vi "SSC Relay Control Single Action Single Site.vi"(0 "SSC Relay in":T1[](array[typedef]), 1 "Site":i32, 5 "Relay Action":T3=21 items=["Open Relay"=20, "Close Relay"=21], 7 "Settling Time (s)":dbl format="%#_12p", 9 "Sites":i32[](array[numeric]), 11 "error in":errorcluster) -> (4 "SSC Relay out":T1[](array[typedef]), 8 "Completed Relay Operations":T2[](array[typedef]) {"Desired State" items=["Open Relay"=20, "Close Relay"=21]}, 15 "error out":errorcluster)   [LabVIEW 2019]
doc: "Performs the specified relay action on all Relays associated with the specified site that are configured in the SSC Relay session. The function will then wait a specified amount of time if the Settling Time (s) input is wired."
uses:
  SSC Relay.ctl
  <instrlib>/niSwitch/niSwitch.llb/niSwitch Relay Action.ctl
  SubVIs/TSM Relay Completed Operations.ctl
  SSC Relay Control Core.vi
  Single SSC Relay NI-Switch Control.vi
  Single SSC Relay Fill Additional Error info.vi
  SSC Relay Expand Action Array to All Sessions.vi
  <vilib>/Utility/error.llb/Error Cluster From Error Code.vi
  <instrlib>/niSwitch/niSwitch.llb/niSwitch Get Relay Position.vi
  <instrlib>/niSwitch/niSwitch.llb/niSwitch Relay Control.vi
  <vilib>/Utility/High Resolution Polling Wait.vi
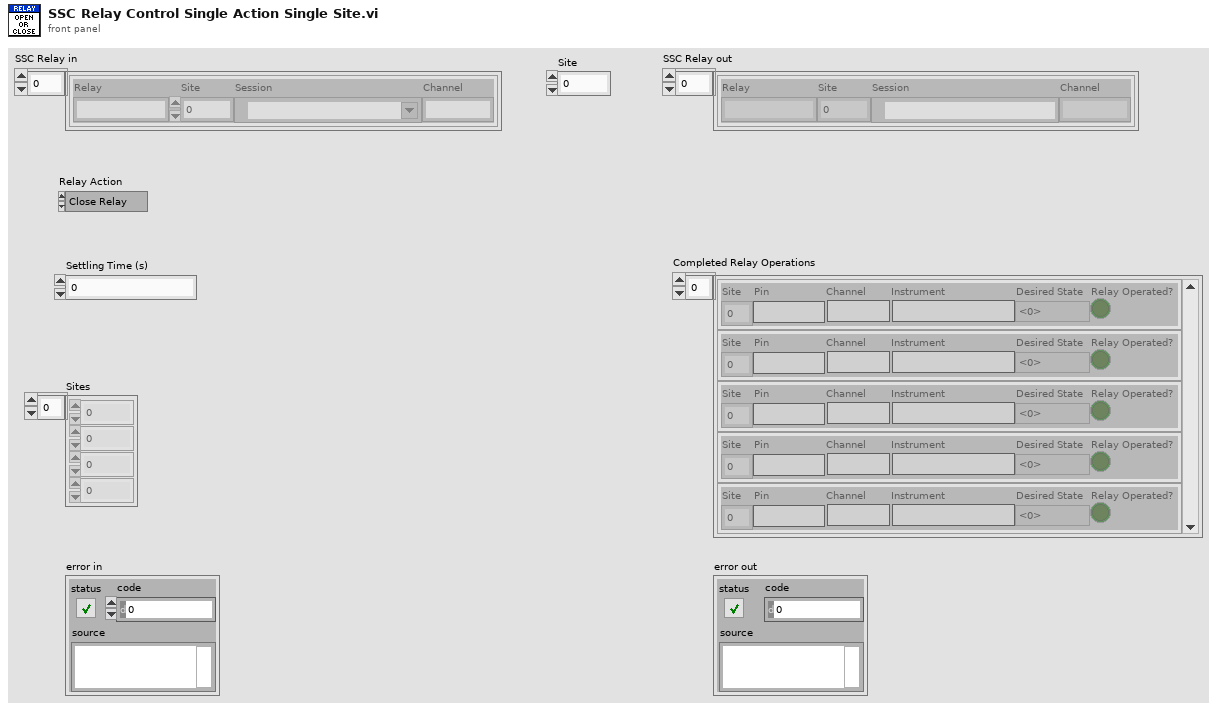
[diagram p1: front panel]
types:
  T1 = typedef "SSC Relay.ctl" = cluster{"Relay":string, "Site":i32, "Session":refnum<k15>, "Channel":string}
  T2 = typedef "TSM Relay Completed Operations.ctl" = cluster{"Site":i32, "Pin":string, "Channel":string, "Instrument":string, "Desired State":T3, "Relay Operated?":bool}
  T3 = typedef "niSwitch Relay Action.ctl" = i32
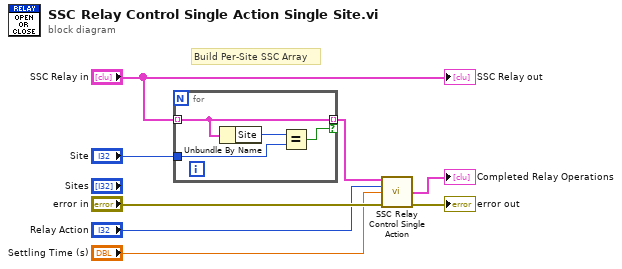
[diagram p0: block diagram]
diagram:
  # "Build Per-Site SSC Array"
  n1 = for {
    tunnel: "SSC Relay in" -> [w12] mode=indexing
    tunnel: [w12] -> w3 mode=indexing if=w10
    tunnel: "Site" -> [w9]
    n2 = Unbundle By Name(w12) -> ("Site"=w11:i32)
    n3 = Equal?(x=w11, y=w9) -> (x = y?=w10:bool)
  }
  n4 = call "SSC Relay Control Single Action.vi"("SSC Relay in"=w3, "Relay Action"="Relay Action", "Settling Time (s)"="Settling Time (s)", "error in"="error in") -> ("Completed Relay Operations"=→"Completed Relay Operations":T2[], "error out"=→"error out":errorcluster)  [unwired: 9 in, 1 out]
  "SSC Relay out" <- "SSC Relay in"
